vi "Get accelaration.vi"(0 "Zaber":T1={"Serial port handle"="", "Axis"="", "Controller #"=0, "Min position"=0.0, "Max position"=0.0, "Min velocity"=0.0, "Max velocity"=0.0, "Firmware"="", "Device ID"=0, "Variable event"=refnum, "Variable ref"=refnum, "Resolution, usteps/step"=0, "Serial port semaphore"=refnum, "Joystick buttons"={"MinDir"=1, "MaxDir"=2, "MedSpeed"=5, "HighSpeed"=6}} {"Joystick buttons"."HighSpeed" min=1 max=25 step=1; "Joystick buttons"."MedSpeed" min=1 max=25 step=1; "Joystick buttons"."MaxDir" min=1 max=25 step=1; "Joystick buttons"."MinDir" min=1 max=25 step=1}, 5 "error in":errorcluster) -> (14 "Zaber out":T1={"Serial port handle"="", "Axis"="", "Controller #"=0, "Min position"=0.0, "Max position"=0.0, "Min velocity"=0.0, "Max velocity"=0.0, "Firmware"="", "Device ID"=0, "Variable event"=refnum, "Variable ref"=refnum, "Resolution, usteps/step"=0, "Serial port semaphore"=refnum, "Joystick buttons"={"MinDir"=1, "MaxDir"=2, "MedSpeed"=5, "HighSpeed"=6}} {"Joystick buttons"."HighSpeed" min=1 max=25 step=1; "Joystick buttons"."MedSpeed" min=1 max=25 step=1; "Joystick buttons"."MaxDir" min=1 max=25 step=1; "Joystick buttons"."MinDir" min=1 max=25 step=1}, 16 "Accelaration, mm/s/s":dbl, 17 "Accelaration, counts":i32, 19 "error out":errorcluster)   [LabVIEW 2018]
uses:
  Zaber.ctl
  GenericDataEvent/GenericEvent.ctl
  ZaberVariables.ctl
  CommandZaber.ctl
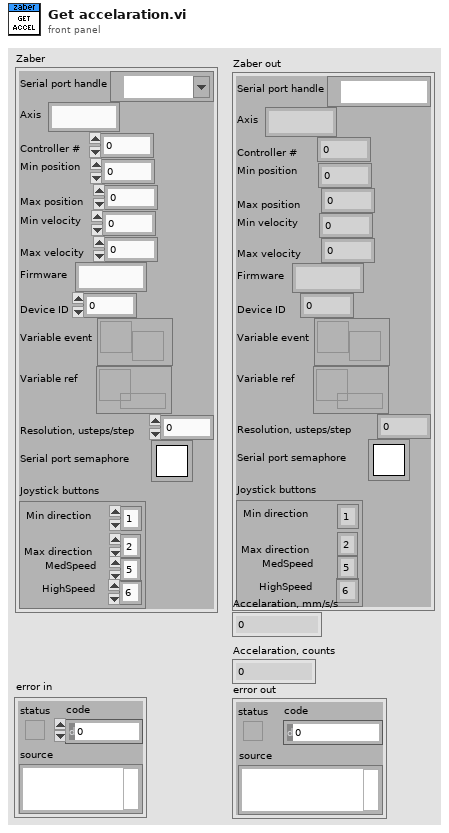
[diagram p1: front panel]
types:
  T1 = typedef "Zaber.ctl" = cluster{"Serial port handle":refnum<visa-resource-name>, "Axis":string, "Controller #":u8, "Min position":dbl, "Max position":dbl, "Min velocity":dbl, "Max velocity":dbl, "Firmware":string, "Device ID":i32, "Variable event":T2, "Variable ref":refnum<data-value>, "Resolution, usteps/step":i32, "Serial port semaphore":T3, "Joystick buttons":cluster{"MinDir":i32, "MaxDir":i32, "MedSpeed":i32, "HighSpeed":i32}}
  T2 = typedef "GenericEvent.ctl" = refnum<user-event>
  T3 = typedef "Semaphore RefNum" = refnum<k1>
  T4 = typedef "CommandZaber.ctl" = cluster{"Command":u8, "Data":i32}
  T5 = typedef "ZaberVariables.ctl" = cluster{"Position":i32, "Speed":i32, "Min soft position":dbl, "Max soft position":dbl, "Accelaration":i32}
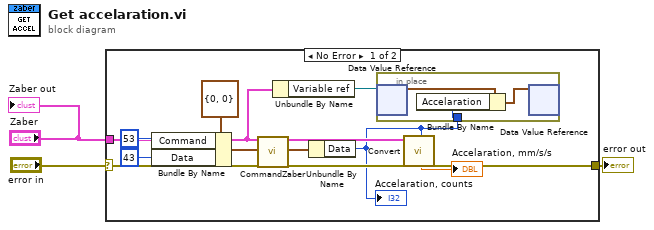
[diagram p0: block diagram]
diagram:
  n1 = case shown="No Error" "error in" {
    selector: "error in" -> [w10 w19]
    tunnel: [w9 w19] -> w2
    tunnel: "Zaber" -> [w6 _]
    frame No Error {
      n2 = Bundle By Name(cluster=T4 {"Command"=0, "Data"=0} ("Command"), "Command"=53 ("Data"), "Data"=43) -> (w14:T4)
      n3 = call "CommandZaber.vi"("Zaber"=w6, "Command"=w14, "error in"=w10) -> ("Zaber out"=w8:T1, "Answer"=w11:T4, "error out"=w9:errorcluster)  [unwired: 13 in, 1 out]
      n4 = Unbundle By Name(w6) -> ("Variable ref"=w5:refnum<data-value>)
      n5 = Unbundle By Name(w11) -> ("Data"=w4:i32)
      "Accelaration, counts" <- w4
      n6 = in-place {
        in-place-border: w4 -> [w16]
        n7 = in-place-dvr #1(w5) -> (w17:T5)  [unwired: 1 out]
        n8 = Bundle By Name(cluster=w17, "Accelaration"=w16) -> (w18:T5)
        n9 = in-place-dvr #1(w18) -> ()  [unwired: 2 out]
      }
      n10 = call "Convert.vi"("Zaber"=w8, "Accelaration, counts"=w4) -> ("Accelaration, mm/s/s"=→"Accelaration, mm/s/s":dbl)  [unwired: 9 in, 8 out]
    }
    frame Error {
    }
  }
  "error out" <- w2
  "Zaber out" <- "Zaber"
